vi "Compare file to FTP directory.vi"(0 "File Management":T1, 1 "FTP Creds":T3={"Host"="", "UserName"="", "PassWord"="", "FTP File Path"="", "FTP Timeout (S)"=60, "Active or Passive"=FALSE, "ASCII or Binary"=FALSE} {"FTP Timeout (S)" min=0 max=300 step=1}, 3 "File output directories":T2={"Archive Location"=path "", "Archive Location 2"=path "<Not A Path>", "OutPut Path"=path "", "Directory(s) To Scan Files"=[]}, 4 "Unmanaged Files Queue":refnum<queue>, 5 "Unmanaged files queue error":errorcluster) -> (14 "number of unmached files":i32, 16 "unmatched file names":string, 18 "Unmanaged Files Queue out":refnum<queue>, 19 "Unmanaged files queue error out":errorcluster)   [LabVIEW 2011]
uses:
  Controls/FTP Credintials.ctl
  Controls/File Path directories.ctl
  Controls/File Management.ctl
panel:
  # "File Handling Method"
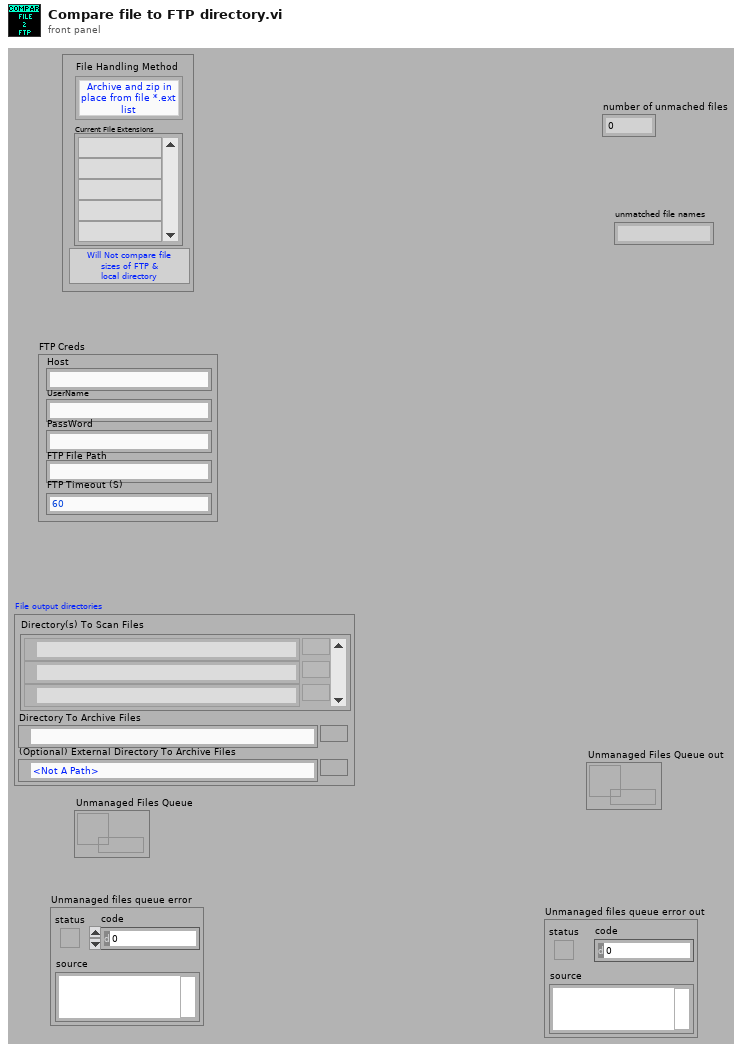
[diagram p1: front panel]
types:
  T1 = typedef "File Management.ctl" = cluster{"Comp File Size":bool, "File Handle Method":enum16{"Archive and zip in place from file *.ext list", "Archive and zip ALL file Types to archive directory", "Archive and zip to archive directory from file *.ext list", "Perform no file management"}, "file extention list":string[]}
  T2 = typedef "File Path directories.ctl" = cluster{"Archive Location":path, "Archive Location 2":path, "OutPut Path":path, "Directory(s) To Scan Files":path[]}
  T3 = typedef "FTP Credintials.ctl" = cluster{"Host":string, "UserName":string, "PassWord":string, "FTP File Path":string, "FTP Timeout (S)":i32, "Active or Passive":bool, "ASCII or Binary":bool}
  T4 = enum16{"Archive and zip in place from file *.ext list", "Archive and zip ALL file Types to archive directory", "Archive and zip to archive directory from file *.ext list", "Perform no file management"}
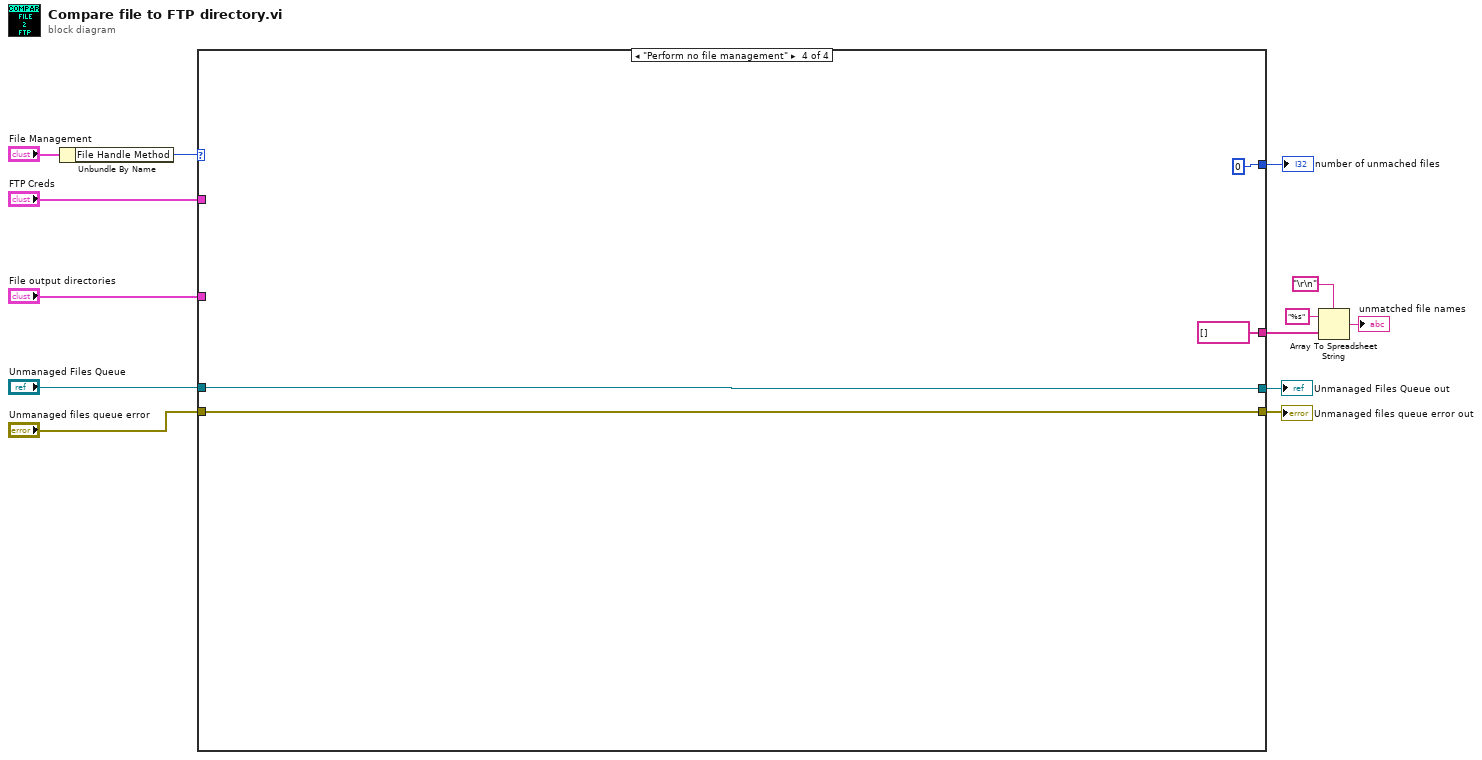
[diagram p0: block diagram]
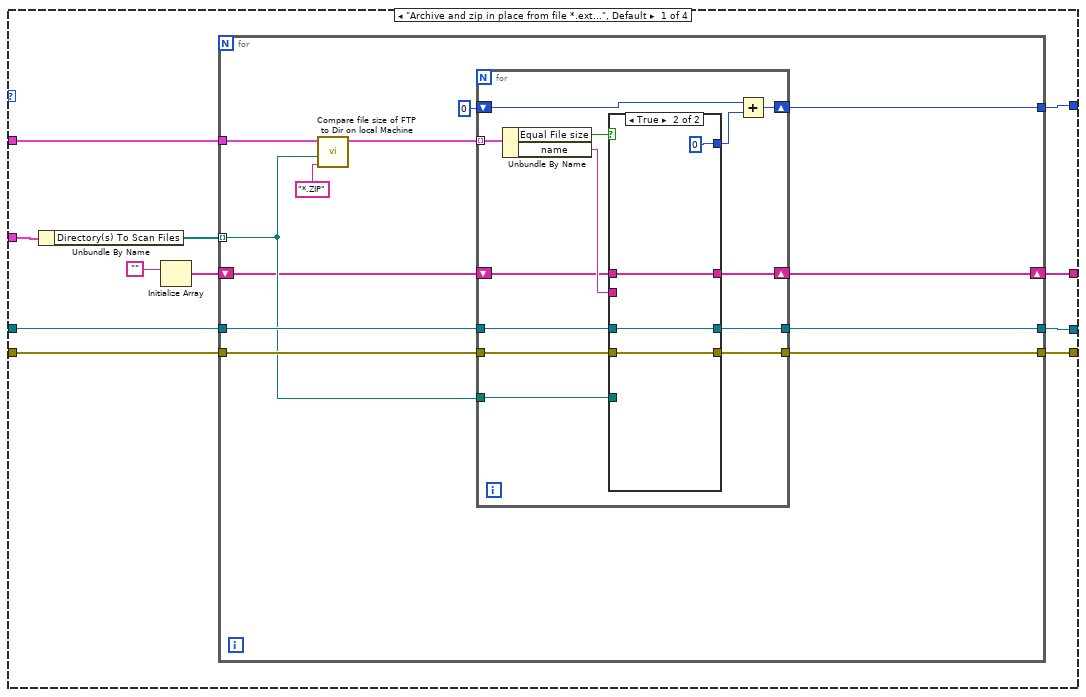
[diagram p2: hidden frame]
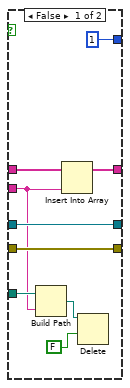
[diagram p3: hidden frame]
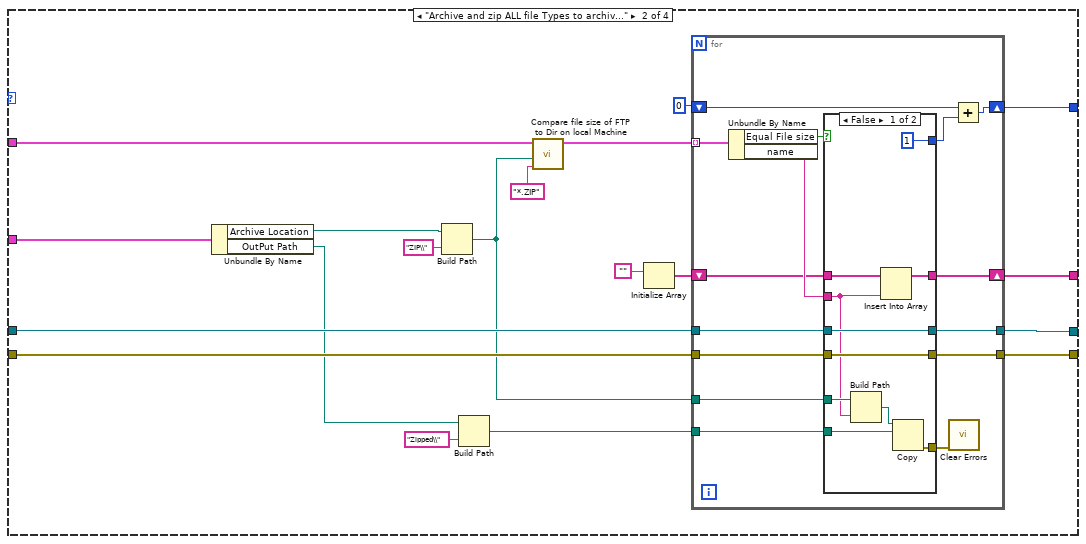
[diagram p4: hidden frame]
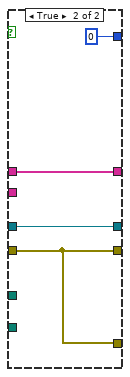
[diagram p5: hidden frame]
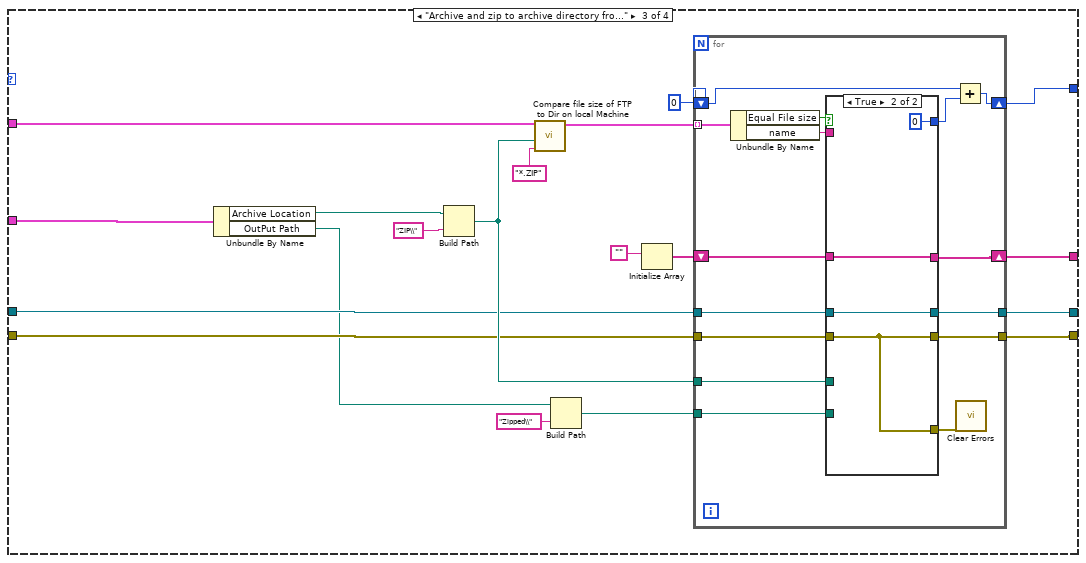
[diagram p6: hidden frame]
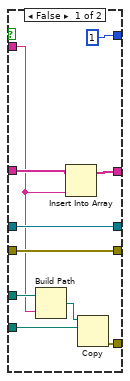
[diagram p7: hidden frame]
diagram:
  n1 = Unbundle By Name("File Management") -> ("File Handle Method"=w5:T4)
  n2 = case shown="\"Perform no file management\"" w5 {
    tunnel: "FTP Creds" -> [w20 w81 w119 _]
    tunnel: "File output directories" -> [w17 w80 w117 _]
    tunnel: "Unmanaged Files Queue" -> [w19 w79 w124 w161]
    tunnel: "Unmanaged files queue error" -> [w18 w78 w123 w162]
    tunnel: [w23 w77 w121 w161] -> w9
    tunnel: [w24 w76 w120 w162] -> w8
    tunnel: [w21 w72 w122 0] -> w7
    tunnel: [w22 w63 w111 string[] []] -> w4
    frame "Archive and zip in place from file *.ext list", Default {
      n3 = Unbundle By Name(w17) -> ("Directory(s) To Scan Files"=w16:path[])
      n4 = Initialize Array("") -> (w15:string[])  [unwired: 1 in]
      n5 = for {
        tunnel: [w33] -> w24
        tunnel: [w32] -> w23
        tunnel: [w31] -> w21
        tunnel: w20 -> [w30]
        tunnel: w19 -> [w29]
        tunnel: w18 -> [w28]
        tunnel: w16 -> [w27] mode=indexing
        shift-right: [w25] -> w22
        shift-left: w15 -> [w26]
        n6 = call "Compare file size of FTP to Dir on local Machine.vi"("File Pattern (*.CSV .ddf)"="*.ZIP", "Local Path to compare file sizes to FTP"=w27, "FTP Creds"=w30) -> ("Equal File Sizes"=w35:cluster{"name":string, "Equal File size":bool}[])  [unwired: 8 in]
        n7 = for {
          tunnel: [w49] -> w32
          tunnel: [w48] -> w33
          tunnel: w29 -> [w46]
          tunnel: w28 -> [w47]
          tunnel: w35 -> [w45] mode=indexing
          shift-right: [w41] -> w31
          shift-left: 0 -> [w40]
          tunnel: w27 -> [w39]
          shift-right: [w37] -> w25
          shift-left: w26 -> [w38]
          n8 = Unbundle By Name(w45) -> ("Equal File size"=w44:bool, "name"=w43:string)
          n9 = case shown="True" w44 {
            tunnel: [w54 w62] -> w49
            tunnel: [w53 w61] -> w48
            tunnel: w47 -> [w53 w61]
            tunnel: w46 -> [w54 w62]
            tunnel: w43 -> [w50 _]
            tunnel: [1 0] -> w42
            tunnel: w39 -> [w56 _]
            tunnel: w38 -> [w52 w59]
            tunnel: [w51 w59] -> w37
            frame False {
              n10 = Build Path(base path=w56, name or relative path=w50) -> (appended path=w57:path)
              n11 = Insert Into Array(array=w52, new element=w50) -> (w51:string[])  [unwired: 1 in]
              n12 = Delete(path (use dialog)=w57, confirm (F)=FALSE ("overwrite (F)")) -> ()  [unwired: 3 in, 3 out]
            }
            frame True {
            }
          }
          n13 = Add(x=w40, y=w42) -> (x+y=w41:i32)
        }
      }
    }
    frame "Archive and zip ALL file Types to archive directory" {
      n14 = Unbundle By Name(w80) -> ("Archive Location"=w70:path, "OutPut Path"=w67:path)
      n15 = Build Path(base path=w70, name or relative path="ZIP\\") -> (appended path=w69:path)
      n16 = Build Path(base path=w67, name or relative path="Zipped\\") -> (appended path=w66:path)
      n17 = call "Compare file size of FTP to Dir on local Machine.vi"("File Pattern (*.CSV .ddf)"="*.ZIP", "Local Path to compare file sizes to FTP"=w69, "FTP Creds"=w81) -> ("Equal File Sizes"=w74:cluster{"name":string, "Equal File size":bool}[])  [unwired: 8 in]
      n18 = Initialize Array("") -> (w64:string[])  [unwired: 1 in]
      n19 = for {
        tunnel: [w96] -> w77
        tunnel: [w95] -> w76
        tunnel: w79 -> [w93]
        tunnel: w78 -> [w94]
        tunnel: w74 -> [w92] mode=indexing
        shift-right: [w88] -> w72
        shift-left: 0 -> [w87]
        tunnel: w66 -> [w86]
        tunnel: w69 -> [w85]
        shift-right: [w82] -> w63
        shift-left: w64 -> [w83]
        n20 = Unbundle By Name(w92) -> ("Equal File size"=w91:bool, "name"=w90:string)
        n21 = case shown="False" w91 {
          tunnel: [w102 w110] -> w96
          tunnel: [w101 w108] -> w95
          tunnel: w94 -> [w101 w108]
          tunnel: w93 -> [w102 w110]
          tunnel: w90 -> [w97 _]
          tunnel: [1 0] -> w89
          tunnel: w86 -> [w105 _]
          tunnel: w85 -> [w103 _]
          tunnel: [w100 w108] -> w84
          tunnel: w83 -> [w99 w107]
          tunnel: [w98 w107] -> w82
          frame False {
            n22 = Build Path(base path=w103, name or relative path=w97) -> (appended path=w104:path)
            n23 = Insert Into Array(array=w99, new element=w97) -> (w98:string[])  [unwired: 1 in]
            n24 = Copy(10:w105, 11:w104) -> (0:w100:errorcluster)  [unwired: 3 in, 2 out]
          }
          frame True {
          }
        }
        n25 = call <vilib>:"Clear Errors.vi"("error in (no error)"=w84) -> ()  [unwired: 6 in, 1 out]
        n26 = Add(x=w87, y=w89) -> (x+y=w88:i32)
      }
    }
    frame "Archive and zip to archive directory from file *.ext list" {
      n27 = Unbundle By Name(w117) -> ("Archive Location"=w118:path, "OutPut Path"=w115:path)
      n28 = Build Path(base path=w118, name or relative path="ZIP\\") -> (appended path=w125:path)
      n29 = call "Compare file size of FTP to Dir on local Machine.vi"("File Pattern (*.CSV .ddf)"="*.ZIP", "Local Path to compare file sizes to FTP"=w125, "FTP Creds"=w119) -> ("Equal File Sizes"=w128:cluster{"name":string, "Equal File size":bool}[])  [unwired: 8 in]
      n30 = Build Path(base path=w115, name or relative path="Zipped\\") -> (appended path=w114:path)
      n31 = Initialize Array("") -> (w113:string[])  [unwired: 1 in]
      n32 = for {
        tunnel: [w144] -> w121
        tunnel: [w143] -> w120
        tunnel: w124 -> [w141]
        tunnel: w123 -> [w142]
        tunnel: w128 -> [w140] mode=indexing
        shift-right: [w136] -> w122
        shift-left: 0 -> [w135]
        tunnel: w125 -> [w134]
        tunnel: w114 -> [w133]
        shift-right: [w130] -> w111
        shift-left: w113 -> [w131]
        n33 = Unbundle By Name(w140) -> ("Equal File size"=w139:bool, "name"=w138:string)
        n34 = case shown="True" w139 {
          tunnel: [w150 w158] -> w144
          tunnel: [w149 w157] -> w143
          tunnel: w142 -> [w149 w157]
          tunnel: w141 -> [w150 w158]
          tunnel: w138 -> [w145 _]
          tunnel: [1 0] -> w137
          tunnel: w134 -> [w152 _]
          tunnel: w133 -> [w151 _]
          tunnel: [w148 w157] -> w132
          tunnel: w131 -> [w147 w155]
          tunnel: [w146 w155] -> w130
          frame False {
            n35 = Build Path(base path=w152, name or relative path=w145) -> (appended path=w153:path)
            n36 = Insert Into Array(array=w147, new element=w145) -> (w146:string[])  [unwired: 1 in]
            n37 = Copy(10:w151, 11:w153) -> (0:w148:errorcluster)  [unwired: 3 in, 2 out]
          }
          frame True {
          }
        }
        n38 = Add(x=w135, y=w137) -> (x+y=w136:i32)
        n39 = call <vilib>:"Clear Errors.vi"("error in (no error)"=w132) -> ()  [unwired: 6 in, 1 out]
      }
    }
    frame "Perform no file management" {
    }
  }
  "Unmanaged Files Queue out" <- w9
  "Unmanaged files queue error out" <- w8
  "number of unmached files" <- w7
  n40 = Array To Spreadsheet String(delimiter (Tab)="\r\n", array=w4, 3:"%s" ("format string")) -> (spreadsheet string=→"unmatched file names":string)
